vi "fileNameToDate.vi"(11 "Sisend":string[](array[string])) -> (3 "V2ljund":string[](array[string]))   [LabVIEW 2012]
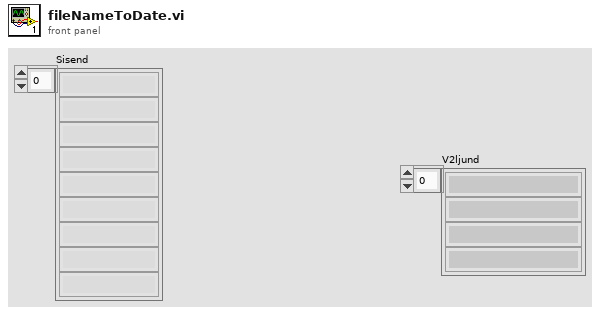
[diagram p1: front panel]
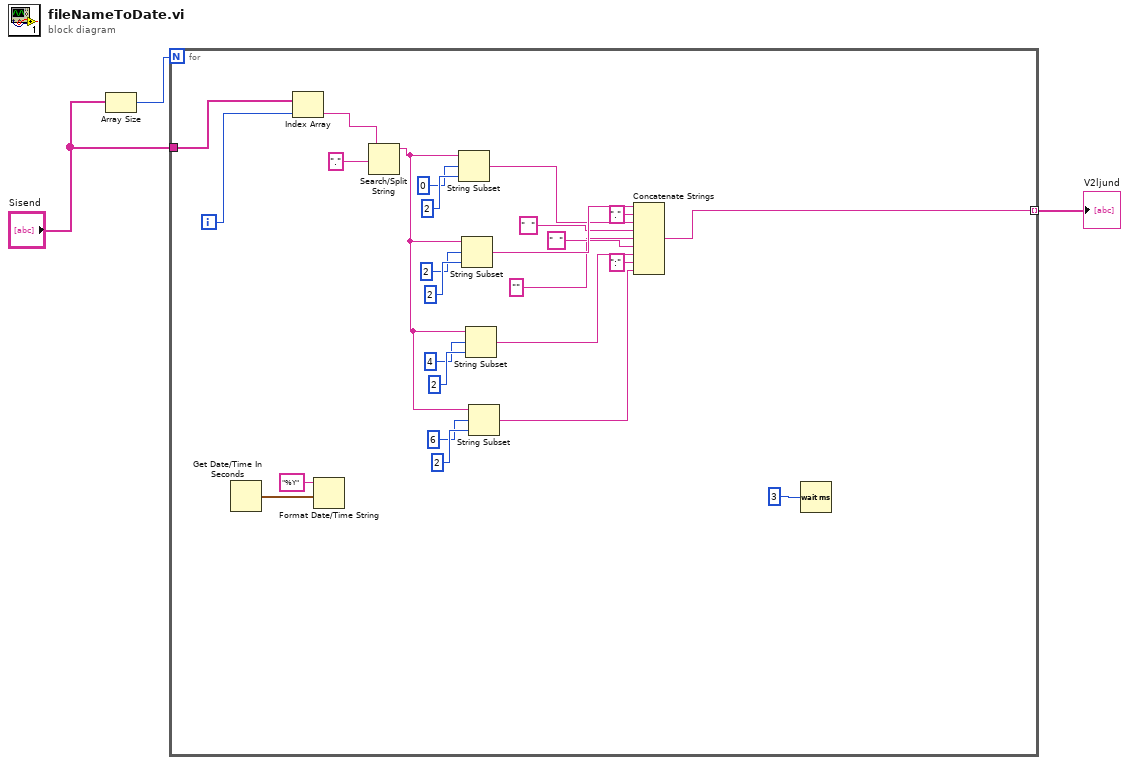
[diagram p0: block diagram]
diagram:
  n1 = Array Size(array="Sisend") -> (size(s)=w1:i32)
  n2 = for {
    N: w1 -> [_]
    tunnel: "Sisend" -> [w26]
    tunnel: [w6] -> w2 mode=indexing
    i -> [w27]
    n3 = Get Date/Time In Seconds() -> (seconds since 1Jan1904=w13:timestamp)
    n4 = Index Array(array=w26, index=w27) -> (element=w28:string)
    n5 = Format Date/Time String(time format string (%c)="%Y", seconds (now)=w13) -> ()  [unwired: 1 in, 1 out]
    n6 = Search/Split String(string=w28, search string/char (-)=".") -> (substring before match=w17:string)  [unwired: 1 in, 2 out]
    n7 = String Subset(string=w17, offset (0)=0, length (rest)=2 ("length (rest)")) -> (substring=w15:string)
    n8 = String Subset(string=w17, offset (0)=2, length (rest)=2 ("length (rest)")) -> (substring=w16:string)
    n9 = String Subset(string=w17, offset (0)=4, length (rest)=2 ("length (rest)")) -> (substring=w9:string)
    n10 = String Subset(string=w17, offset (0)=6, length (rest)=2 ("length (rest)")) -> (substring=w7:string)
    n11 = Concatenate Strings(w16, "." ("string"), w15, "  " ("string"), "" ("string"), "  " ("string"), w9, ":" ("string"), w7) -> (w6:string)
    n12 = Wait (ms)(milliseconds to wait=u32 3 ("delay kuupäev")) -> ()  [unwired: 1 out]
  }
  "V2ljund" <- w2
